vi "HIOKI PW3390 Meas Integ State.vi"(0 "VISA Resource":refnum<visa-resource-name>, 11 "error in (no error)":errorcluster) -> (4 "VISA Resource out":refnum<visa-resource-name>, 6 "State out":enum16{"RESET", "STOP", "WAIT", "RUN"}(ring), 15 "error out":errorcluster)   [LabVIEW 2009]
doc: "State out\n Outputs the query results of the device's integration status."
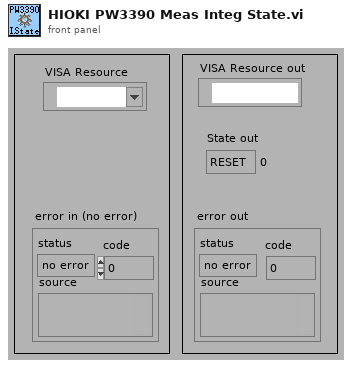
[diagram p1: front panel]
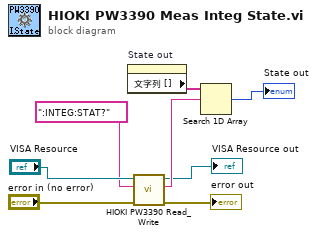
[diagram p0: block diagram]
diagram:
  n1 = property on="State out" class="Enum (strict)"() -> ("文字列 []"=w3:string[])  [unwired: 2 in, 2 out]
  n2 = call <instrlib>:"HIOKI PW3390 Read_Write.vi"("error in (no error)"="error in (no error)", "data in"=":INTEG:STAT?", "VISA Resource"="VISA Resource") -> ("error out"=→"error out":errorcluster, "data out"=w4:string, "VISA Resource out"=→"VISA Resource out":refnum<visa-resource-name>)  [unwired: 6 in]
  n3 = Search 1D Array(1D array=w3, element=w4) -> (index of element=→"State out":i32)  [unwired: 1 in]
